vi "Initialize From Settings.vi"(8 "error in (no error)":errorcluster, 10 "settings":cluster{"key":string, "value":string}[](array[cluster]), 11 "Thread Configuration in":refnum<class "Thread Configuration.lvclass">) -> (0 "error out":errorcluster, 3 "Thread Configuration out":refnum<class "Thread Configuration.lvclass">)   [LabVIEW 2017, in "GE Reflective Memory.lvlib" / "Thread Configuration.lvclass"]
uses:
  Thread Configuration.lvclass
  Thread Configuration.lvclass/Thread Configuration.ctl
  Driver/Source/Typedefs/GE 5565PIORC.Typedef.DMA Wait Mode.ctl
  GE Reflective Memory.lvlib
  Driver/Source/GE 5565PIORC.lvclass
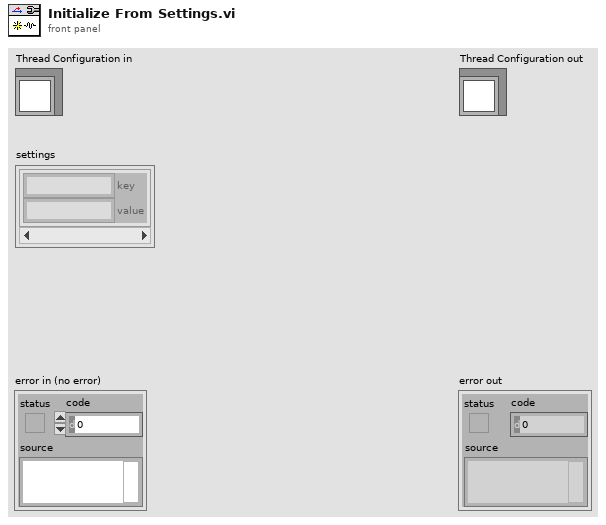
[diagram p1: front panel]
types:
  T1 = typedef "GE 5565PIORC.lvclass/GE 5565PIORC.Typedef.DMA Wait Mode.ctl" = enum16{"Polling", "Interrupt"}
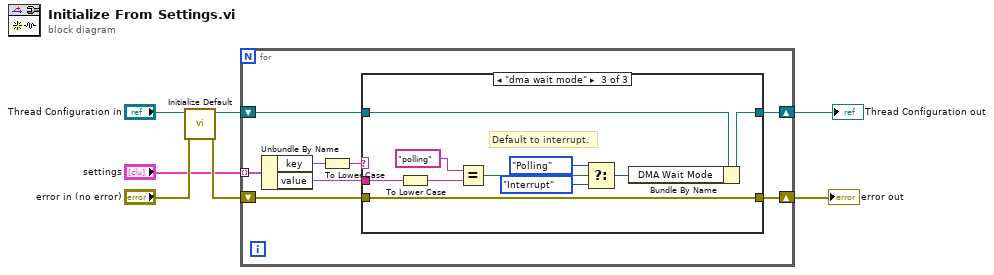
[diagram p0: block diagram]
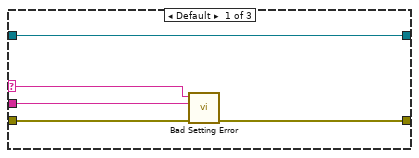
[diagram p2: hidden frame]
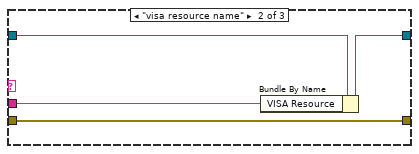
[diagram p3: hidden frame]
diagram:
  n1 = call-dynamic "Initialize Default.vi"("error in (no error)"="error in (no error)", "Thread Configuration in"="Thread Configuration in") -> ("error out"=w2:errorcluster, "Thread Configuration out"=w4:refnum<class "Thread Configuration.lvclass">)  [unwired: 8 in]
  n2 = for {
    shift-right: [w9] -> w7
    shift-left: w2 -> [w10]
    tunnel: "settings" -> [w15] mode=indexing
    shift-right: [w11] -> w6
    shift-left: w4 -> [w12]
    n3 = Unbundle By Name(w15) -> ("key"=w14:string, "value"=w8:string)
    n4 = To Lower Case(string=w14) -> (all lower case string=w13:string)
    n5 = case shown="\"dma wait mode\"" w13 {
      selector: w13 -> [w17 _ _]
      tunnel: w8 -> [w16 w21 w31]
      tunnel: w12 -> [w18 w24 w34]
      tunnel: [w18 w23 w33] -> w11
      tunnel: w10 -> [w20 w22 w32]
      tunnel: [w19 w22 w32] -> w9
      frame Default {
        n6 = call "Bad Setting Error.vi"("error in (no error)"=w20, "value"=w16, "key"=w17) -> ("error out"=w19:errorcluster)  [unwired: 8 in]
      }
      frame "visa resource name" {
        n7 = Bundle By Name(cluster=w24, "VISA Resource"=w21) -> (w23:refnum<class "Thread Configuration.lvclass">)
      }
      frame "dma wait mode" {
        # "Default to interrupt."
        n8 = To Lower Case(string=w31) -> (all lower case string=w25:string)
        n9 = Equal?(x="polling" ("y"), y=w25) -> (x = y?=w29:bool)
        n10 = Select(t=GE_5565PIORC.Typedef.DMA_Wait_Mode."Polling" ("DMA Wait Mode"), s=w29, f=GE_5565PIORC.Typedef.DMA_Wait_Mode."Interrupt" ("DMA Wait Mode")) -> (s? t:f=w28:T1)
        n11 = Bundle By Name(cluster=w34, "DMA Wait Mode"=w28) -> (w33:refnum<class "Thread Configuration.lvclass">)
      }
    }
  }
  "error out" <- w7
  "Thread Configuration out" <- w6
